vi "GyrotoDegree.vi"(1 "GyroDevRef":T1) -> (0 "Delta Degree":dbl format="%.2f")   [LabVIEW 2013]
uses:
  <vilib>/Rock Robotics/WPI/Gyro/WPI_GyroDevRef.ctl
  <vilib>/Rock Robotics/SystemInterfaces/Typedef/FPGA_TypedefAnalogModule.ctl
  <vilib>/Rock Robotics/SystemInterfaces/AI/FPGA_AIChannel.ctl
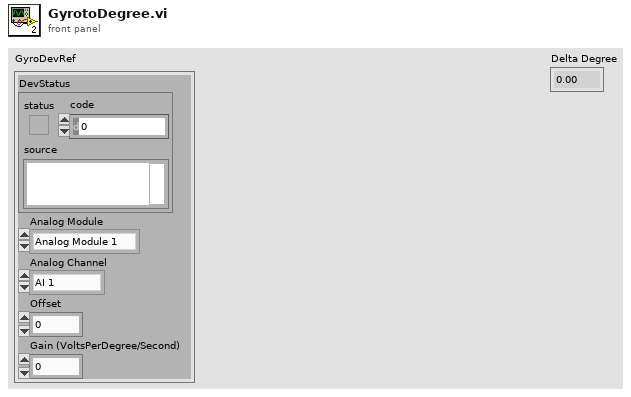
[diagram p1: front panel]
types:
  T1 = typedef "WPI_GyroDevRef.ctl" = cluster{"DevStatus":errorcluster, "Analog Module":T2, "Analog Channel":T3, "Offset":dbl, "Gain (VoltsPerDegree/Second)":dbl}
  T2 = typedef "FPGA_TypedefAnalogModule.ctl" = enum16{"Analog Module 1", "Analog Module 2"}
  T3 = typedef "FPGA_AIChannel.ctl" = enum8{"AI 1", "AI 2", "AI 3", "AI 4", "AI 5", "AI 6", "AI 7", "AI 8", "Invalid"}
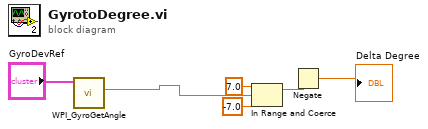
[diagram p0: block diagram]
diagram:
  n1 = call <vilib>:"WPI_GyroGetAngle.vi"("GyroDevRef"="GyroDevRef") -> ("Angle"=w2:dbl)  [unwired: 7 in, 3 out]
  n2 = In Range and Coerce(upper limit=7.0, x=w2, lower limit=-7.0) -> (coerced(x)=w4:dbl)  [unwired: 1 out]
  n3 = Negate(x=w4) -> (-x=→"Delta Degree":dbl)
